vi "ControlToCommandMulti.vi"(10 "SetGetCommands":string, 11 "Control Array":refnum<vi>[](array[refnum])) -> (3 "ControlToCommand":map{refnum<vi>, string[]}(c390))   [LabVIEW 2019, in "TextControlledInstrum.lvlib"]
uses:
  TextControlledInstrum.lvlib
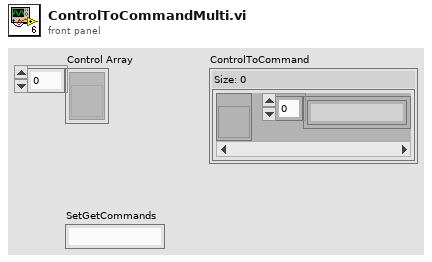
[diagram p1: front panel]
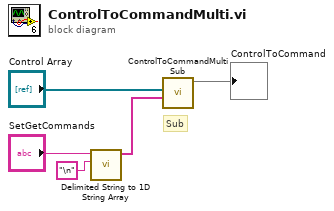
[diagram p0: block diagram]
diagram:
  # "Sub"
  n1 = call <vilib>:"Delimited String to 1D String Array.vi"("delimiter"="\n", "delimited string"="SetGetCommands") -> ("string array"=w2:string[])  [unwired: 9 in]
  n2 = call "ControlToCommandMultiSub.vi"("Command Array"=w2, "Control Array"="Control Array") -> ("ControlToCommand out"=→"ControlToCommand":map{refnum<vi>, string[]})  [unwired: 8 in, 1 out]
